vi "Get Overrides.vi"(6 "timeout (ms)":i32=5000, 8 "error in":errorcluster, 11 "gRPC ID":T3) -> (0 "error out":errorcluster, 2 "Plugin Overrides":T1, 3 "gRPC ID out":T3)   [LabVIEW 2021, in "CIFCoreWrapper.lvlib"]
uses:
  CIFCoreWrapper.lvlib
  CIFCorePlugin_client/CIFCorePlugin_client.lvlib
  <vilib>/gRPC/LabVIEW gRPC Library/Shared/grpcId.ctl
  <vilib>/gRPC/LabVIEW gRPC Library/grpc-lvsupport-release.lvlib
  CIFCorePlugin_client/RPC Messages/cif_plugincore_TimingOverrides.ctl
  CIFCorePlugin_client/RPC Messages/cif_plugincore_PluginOverrides.ctl
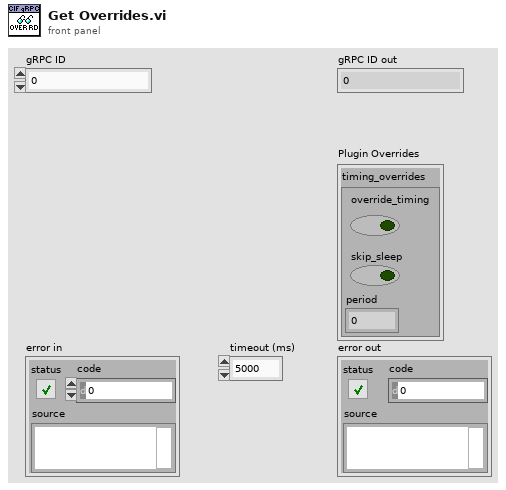
[diagram p1: front panel]
types:
  T1 = typedef "CIFCorePlugin_client.lvlib/cif_plugincore_PluginOverrides.ctl" = cluster{"timing_overrides":T2}
  T2 = typedef "CIFCorePlugin_client.lvlib/cif_plugincore_TimingOverrides.ctl" = cluster{"override_timing":bool, "skip_sleep":bool, "period":dbl}
  T3 = typedef "grpc-lvsupport-release.lvlib/grpcId.ctl" = u64
  T4 = typedef "CIFCorePlugin_client.lvlib/cif_plugincore_GetOverridesResponse.ctl" = cluster{"plugin_overrides":T1}
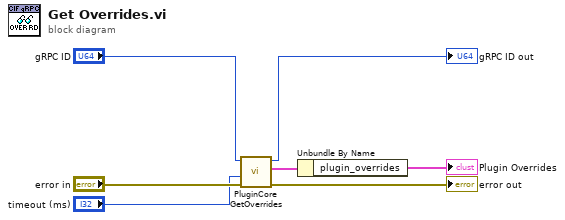
[diagram p0: block diagram]
diagram:
  n1 = call "PluginCore GetOverrides.vi"("error in"="error in", "timeout (ms)"="timeout (ms)", "gRPC ID"="gRPC ID") -> ("error out"=→"error out":errorcluster, "Response Data"=w2:T4, "gRPC ID out"=→"gRPC ID out":T3)  [unwired: 6 in]
  n2 = Unbundle By Name(w2) -> ("plugin_overrides"=→"Plugin Overrides":T1)
